vi "GetType.vi"(0 "reference in":refnum<class "DA.lvclass">) -> (4 "reference out":refnum<class "DA.lvclass">, 6 "obj_type":T1)   [LabVIEW 2019, in "DA.lvclass"]
uses:
  DA.lvclass
  Logger_class/ObjType.ctl
  Logger_class/Logger.lvclass
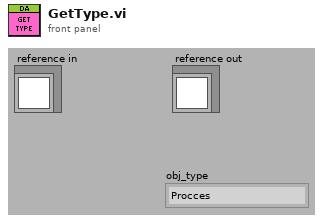
[diagram p1: front panel]
types:
  T1 = typedef "Logger.lvclass/ObjType.ctl" = enum16{"Procces", "Device", "Signal", "DI", "DO", "DA", "AI", "AO", "AA"}
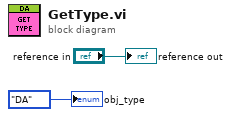
[diagram p0: block diagram]
diagram:
  "reference out" <- "reference in"
  "obj_type" <- ObjType."DA" ("obj_type")
